vi "Stop Core.vi"(10 "final error code":i32, 11 "Nested in":refnum<class "Communicator Worker.lvclass">) -> (3 "Nested out":refnum<class "Communicator Worker.lvclass">)   [LabVIEW 2024, in "Communicator Worker.lvlib" / "Communicator Worker.lvclass"]
doc: "(<B>Filename</B>: Actor Framework.lvlib:Actor.lvclass:Stop Core.vi)\n\nDefines what the actor does before it stops. Use the <B>final error code</B> input to determine whether the actor shut down in response to an error.\n\nBy default, this method does nothing. A descendant class may override it to define behavior, such as shutting down any processes the actor initiated in its override of the Actor Core method."
uses:
  Communicator Worker.lvclass
  Communicator Worker.lvclass/Communicator Worker.ctl
  <vilib>/ActorFramework/Actor/Actor.lvclass
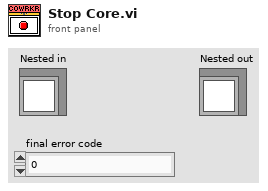
[diagram p1: front panel]
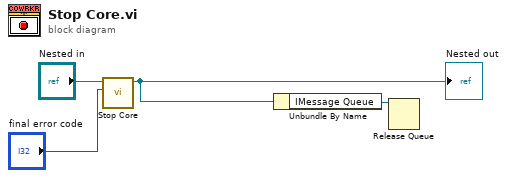
[diagram p0: block diagram]
diagram:
  n1 = call-parent "Stop Core.vi"("final error code"="final error code", "Actor in"="Nested in") -> ("Actor out"=w2:refnum<class "Communicator Worker.lvclass">)  [unwired: 9 in]
  "Nested out" <- w2
  n2 = Unbundle By Name(w2) -> ("IMessage Queue"=w1:refnum<queue>)
  n3 = Release Queue(queue=w1) -> ()  [unwired: 2 in, 3 out]
